vi "AI Init.vi"(7 "ADC #":T1=-1, 8 "error in (no error)":errorcluster, 11 "VisaComms in":refnum<class "VisaComms.lvclass">) -> (0 "error out":errorcluster, 3 "VisaComms out":refnum<class "VisaComms.lvclass">)   [LabVIEW 2020, in "CTI.lvlib" / "VisaComms.lvclass"]
uses:
  VisaComms.lvclass
  ADC Number.ctl
  VisaComms.lvclass/VisaComms.ctl
  Clean Visa Errors.vi
  CTI.lvlib
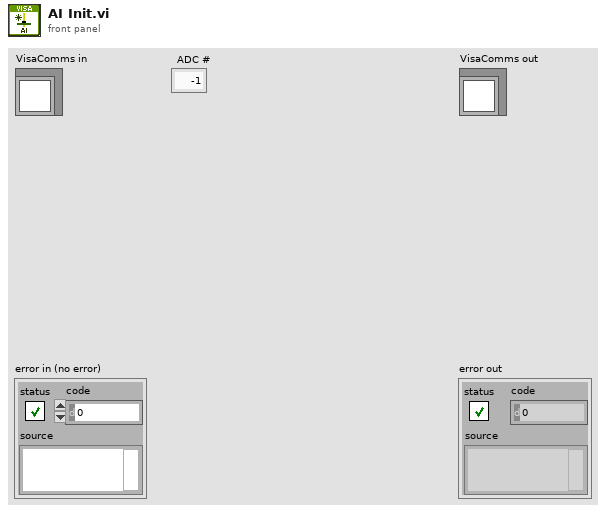
[diagram p1: front panel]
types:
  T1 = typedef "CTI.lvlib/ADC Number.ctl" = i8
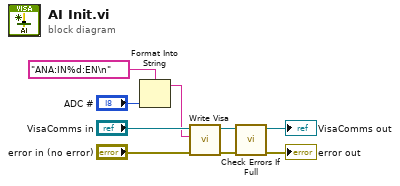
[diagram p0: block diagram]
diagram:
  n1 = Format Into String(format string="ANA:IN%d:EN\n", "ADC #") -> (resulting string=w1:string)  [unwired: 2 in, 1 out]
  n2 = call "Write Visa.vi"("error in (no error)"="error in (no error)", "write buffer"=w1, "VisaComms in"="VisaComms in") -> ("error out"=w3:errorcluster, "VisaComms out"=w4:refnum<class "VisaComms.lvclass">)  [unwired: 6 in, 1 out]
  n3 = call "Check Errors If Full.vi"("error in (no error)"=w3, "VisaComms in"=w4) -> ("error out"=→"error out":errorcluster, "VisaComms out"=→"VisaComms out":refnum<class "VisaComms.lvclass">)  [unwired: 8 in]
